vi "Write Instrument Descriptor.vi"(8 "error in (no error)":errorcluster, 10 "Instrument Descriptor":refnum<k15>="Dev1", 11 "PXI 4070 in":refnum<class "PXI 4070.lvclass">) -> (0 "error out":errorcluster, 3 "PXI 4070 out":refnum<class "PXI 4070.lvclass">)   [LabVIEW 2013, in "PXI 4070.lvclass"]
uses:
  PXI 4070.lvclass
  PXI 4070.lvclass/PXI 4070.ctl
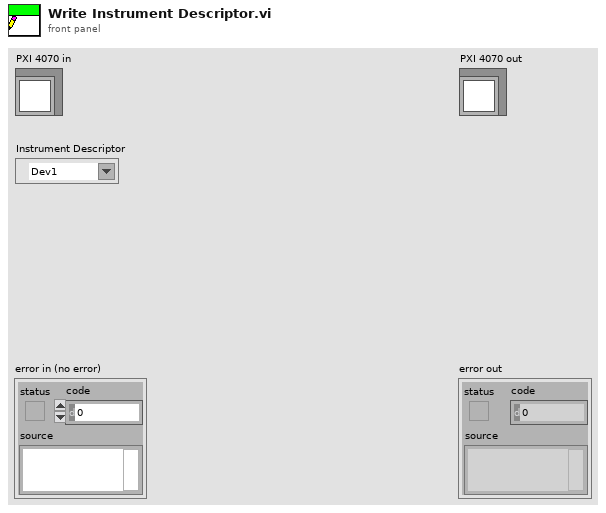
[diagram p1: front panel]
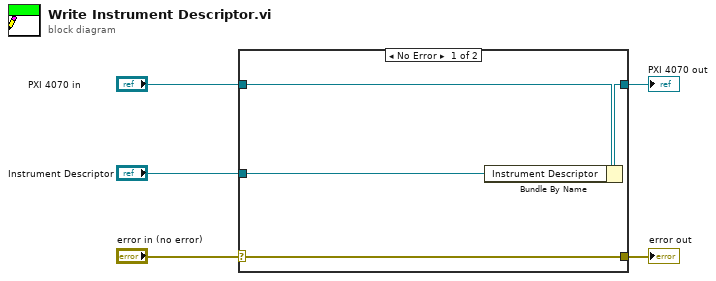
[diagram p0: block diagram]
diagram:
  n1 = case shown="No Error" "error in (no error)" {
    selector: "error in (no error)" -> [w9 w10]
    tunnel: [w9 w10] -> w4
    tunnel: [w7 w11] -> w2
    tunnel: "PXI 4070 in" -> [w8 w11]
    tunnel: "Instrument Descriptor" -> [w6 _]
    frame No Error {
      n2 = Bundle By Name(cluster=w8, "Instrument Descriptor"=w6) -> (w7:refnum<class "PXI 4070.lvclass">)
    }
    frame Error {
    }
  }
  "error out" <- w4
  "PXI 4070 out" <- w2
